vi "STM Read Msg.vi"(7 "Ignore Timeout Error":bool=TRUE, 8 "error in":errorcluster, 9 "Meta data":T1[](array[typedef]), 10 "timeout ms (25000)":i32=25000, 11 "connection ID":refnum<k5>) -> (0 "error out":errorcluster, 1 "Meta element":T1, 2 "data string":string, 3 "connection ID out":refnum<k5>, 4 "Data Size":i32, 5 "Timed Out?":bool)   [LabVIEW 2015]
doc: "This VI reads an incoming package of data from a host. This VI parses the package and extracts the data name and type as described in the meta data.\n\nFor the package to be parsed correctly, the meta data must be consistent in both the sender and the receiver. The data is packaged based on the existing meta data on the sender. \n\nUse the \"Read Meta\" and \"Write Meta\" VIs to ensure that both client and server have the same meta data.\n\nThe data is returned as a string. It is the responsibility of the user to cast it to the appropriate type."
uses:
  Data Def/stm_MetaElement.ctl
  Data Def/stm_MetaDataElement.ctl
  Data Def/stm_MetaID.ctl
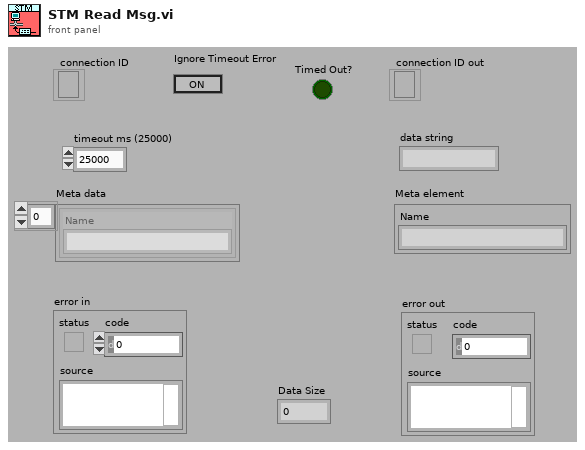
[diagram p1: front panel]
types:
  T1 = typedef "stm_MetaElement.ctl" = cluster{"Name":T2}
  T2 = typedef "stm_MetaDataElement.ctl" = string
  T3 = typedef "stm_MetaID.ctl" = u16
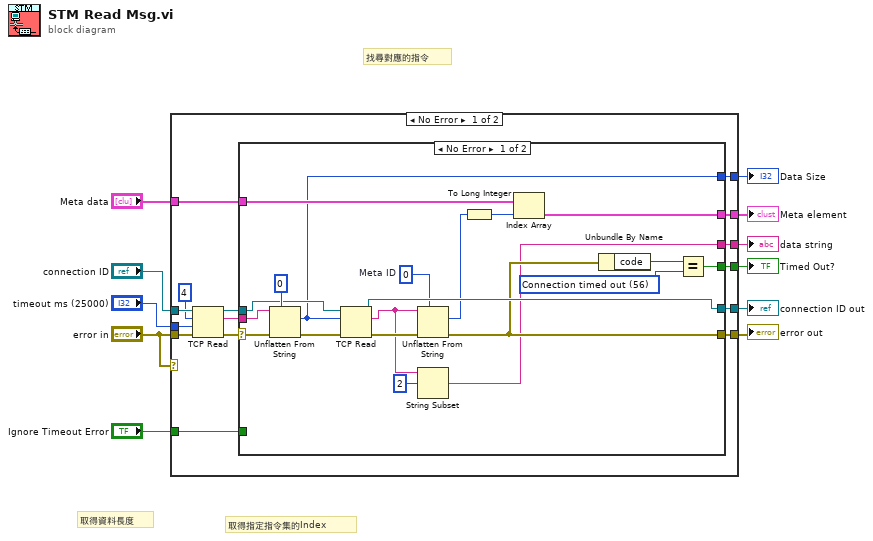
[diagram p0: block diagram]
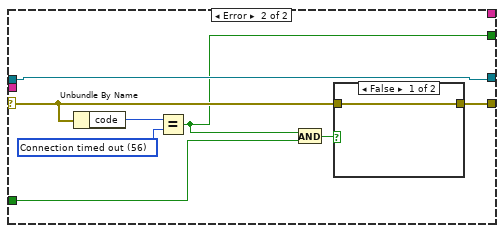
[diagram p2: hidden frame]
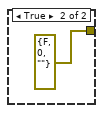
[diagram p3: hidden frame]
diagram:
  # "找尋對應的指令"
  # "取得指定指令集的Index"
  # "取得資料長度"
  n1 = case shown="No Error" "error in" {
    tunnel: "error in" -> [w26 w57]
    tunnel: "connection ID" -> [w25 w58]
    tunnel: "Meta data" -> [w21 _]
    tunnel: "timeout ms (25000)" -> [w20 _]
    tunnel: [w18 w58] -> w8
    tunnel: [w17 w57] -> w7
    tunnel: "Ignore Timeout Error" -> [w16 _]
    tunnel: [w15 _] -> w5
    tunnel: [w14 _] -> w4
    tunnel: [w13 _] -> w3
    tunnel: [w12 _] -> w1
    frame No Error {
      n2 = TCP Read(connection ID=w25, bytes to read=4, error in (no error)=w26, 9:w20) -> (connection ID out=w22:refnum<k5>, data out=w23:string, error out=w19:errorcluster)  [unwired: 1 out]
      n3 = case shown="No Error" w19 {
        selector: w19 -> [w38 w48]
        tunnel: w23 -> [w39 _]
        tunnel: w22 -> [w45 w54]
        tunnel: w21 -> [w44 _]
        tunnel: [w43 w54] -> w18
        tunnel: [w35 w49] -> w17
        tunnel: w16 -> [_ w51]
        tunnel: [w40 w47] -> w15
        tunnel: [w34 _] -> w14
        tunnel: [w29 _] -> w13
        tunnel: [w33 _] -> w12
        frame No Error {
          w32 = T3 0  # Meta ID
          w41 = 56 items=["No Error", "Argument Error", "Memory Full", "Out of Zone", "End of File", "File Already Open", "Generic File IO Error", "File Not Found", "File Permission Error", "Disk Full", "Duplicate Path", "Too Many Files Open", "Not Enabled", "Resource File Not Found", "Cannot Add Resource", "Resource Not Found", "Image Not Found", "Image Memory Error", "Pen Does Not Exist", "Config Bad Type", "Config Token Not Found", "Config Parse Error", "Config Memory Error", "Bad External Code Format", "Bad External Code Offset", "External Code Not Present", "Null Window", "Destroy Window Mixup", "Null Menu", "Print Aborted", "Bad Print Record", "Print Driver Error", "Windows Error During Print", "Memory Error During Print", "Print Dialog Error", "Generic Print Error", "Invalid Device Refnum", "Device Not Found", "Device Parameter Error", "Device Unit Error", "Can't Open Device", "Device Call Aborted", "Generic Error", "Cancelled By User", "Object ID Too Low", "Object ID Too High", "Object Not In Heap", "Unknown Heap", "Bad DefProc ID", "DefProc Not In Table", "Message Out Of Range", "Null Method", "Unknown Message", "Manager Call Not Supported", "Bad address", "Connection In progress", "Connection timed out", "Connection is already in progress", "Network attribute not supported", "Network error", "Address in use", "System out of memory", "Connection aborted", "Connection refused", "Connection is not connected", "Connection is already connected", "Connection closed", "Initialize error (interapplication manager)", "Bad occurrence", "Wait on unbound occurrence handler", "Occurrence queue overflow", "Bad path", "Semaphore not signaled", "Unrecognized type (interapplication manager)"] ("1st Error to Convert")
          n4 = Unflatten From String(type=0 ("bytes to read"), binary string=w39, error in (no error)=w38) -> (value=w33:i32, error out=w37:errorcluster)  [unwired: 1 in, 2 out]
          n5 = TCP Read(connection ID=w45, bytes to read=w33, error in (no error)=w37) -> (connection ID out=w43:refnum<k5>, data out=w30:string, error out=w36:errorcluster)  [unwired: 2 out]
          n6 = Unflatten From String(type=w32, binary string=w30, error in (no error)=w36) -> (value=w28:T3, error out=w35:errorcluster)  [unwired: 3 out]
          n7 = String Subset(string=w30, offset (0)=2) -> (substring=w29:string)  [unwired: 1 out]
          n8 = To Long Integer(number=w28) -> (32bit integer=w27:i32)
          n9 = Index Array(array=w44, index=w27) -> (element=w34:T1)
          n10 = Unbundle By Name(w35) -> ("code"=w42:i32)
          n11 = Equal?(x=w42, y=w41) -> (x = y?=w40:bool)
        }
        frame Error {
          w52 = 56 items=["No Error", "Argument Error", "Memory Full", "Out of Zone", "End of File", "File Already Open", "Generic File IO Error", "File Not Found", "File Permission Error", "Disk Full", "Duplicate Path", "Too Many Files Open", "Not Enabled", "Resource File Not Found", "Cannot Add Resource", "Resource Not Found", "Image Not Found", "Image Memory Error", "Pen Does Not Exist", "Config Bad Type", "Config Token Not Found", "Config Parse Error", "Config Memory Error", "Bad External Code Format", "Bad External Code Offset", "External Code Not Present", "Null Window", "Destroy Window Mixup", "Null Menu", "Print Aborted", "Bad Print Record", "Print Driver Error", "Windows Error During Print", "Memory Error During Print", "Print Dialog Error", "Generic Print Error", "Invalid Device Refnum", "Device Not Found", "Device Parameter Error", "Device Unit Error", "Can't Open Device", "Device Call Aborted", "Generic Error", "Cancelled By User", "Object ID Too Low", "Object ID Too High", "Object Not In Heap", "Unknown Heap", "Bad DefProc ID", "DefProc Not In Table", "Message Out Of Range", "Null Method", "Unknown Message", "Manager Call Not Supported", "Bad address", "Connection In progress", "Connection timed out", "Connection is already in progress", "Network attribute not supported", "Network error", "Address in use", "System out of memory", "Connection aborted", "Connection refused", "Connection is not connected", "Connection is already connected", "Connection closed", "Initialize error (interapplication manager)", "Bad occurrence", "Wait on unbound occurrence handler", "Occurrence queue overflow", "Bad path", "Semaphore not signaled", "Unrecognized type (interapplication manager)"] ("1st Error to Convert")
          n12 = Unbundle By Name(w48) -> ("code"=w53:i32)
          n13 = Equal?(x=w53, y=w52) -> (x = y?=w47:bool)
          n14 = And(x=w47, y=w51) -> (x .and. y?=w50:bool)
          n15 = case shown="False" w50 {
            tunnel: [w55 errorcluster {"status"=FALSE, "code"=0, "source"=""} ("error out")] -> w49
            tunnel: w48 -> [w55 _]
            frame False {
            }
            frame True {
            }
          }
        }
      }
    }
    frame Error {
    }
  }
  "error out" <- w7
  "connection ID out" <- w8
  "Timed Out?" <- w5
  "data string" <- w3
  "Meta element" <- w4
  "Data Size" <- w1
